vi "init.vi"(8 "error in (no error)":errorcluster, 11 "genericVehicle in":refnum<class "genericVehicle.lvclass">) -> (0 "error out":errorcluster, 3 "genericVehicle out":refnum<class "genericVehicle.lvclass">)   [LabVIEW 2011, in "genericVehicle.lvclass"]
uses:
  genericVehicle.lvclass
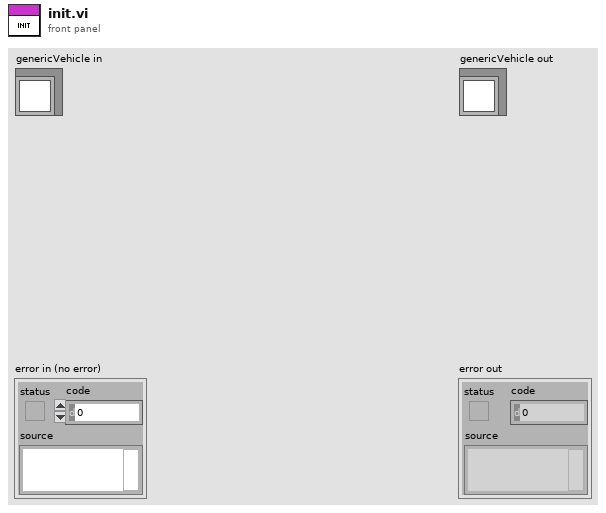
[diagram p1: front panel]
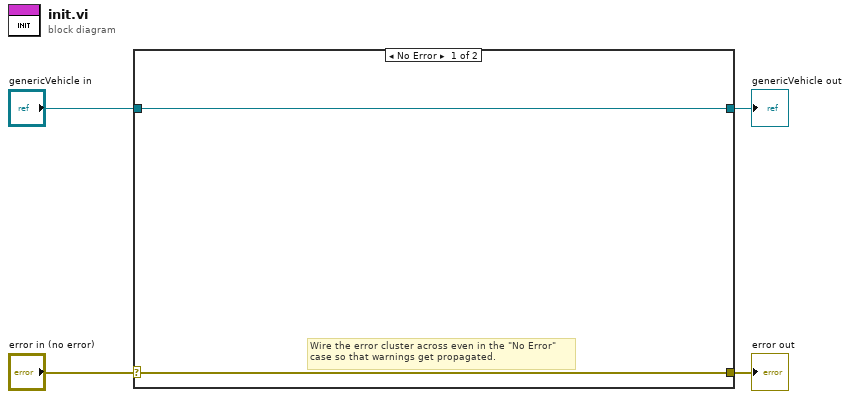
[diagram p0: block diagram]
diagram:
  n1 = case shown="No Error" "error in (no error)" {
    selector: "error in (no error)" -> [w5 w8]
    tunnel: [w5 w8] -> w3
    tunnel: [w6 w7] -> w1
    tunnel: "genericVehicle in" -> [w6 w7]
    frame No Error {
      # "Wire the error cluster across even in the \"No Error\"\ncase so that warnings get propagated."
    }
    frame Error {
    }
  }
  "error out" <- w3
  "genericVehicle out" <- w1
